vi "Local Test.vi"() -> ()   [LabVIEW 2017]
panel:
  out "String 2":string
  out "Dbl 2":dbl
  out "Boolean 2":bool
  in  "String":string
  in  "Dbl":dbl
  in  "Boolean":bool
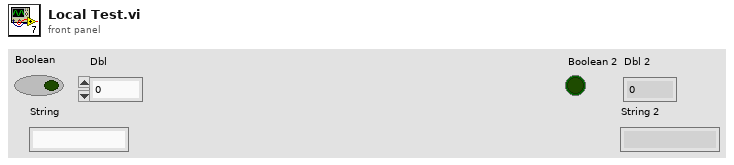
[diagram p1: front panel]
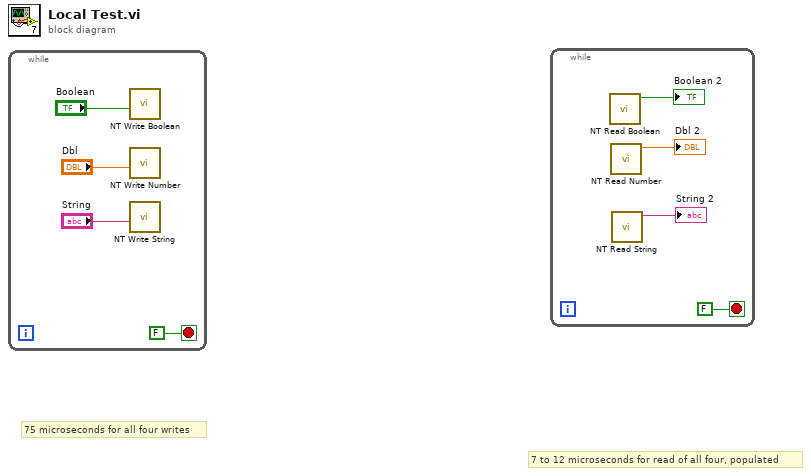
[diagram p0: block diagram]
diagram:
  # "7 to 12 microseconds for read of all four, populated"
  # "75 microseconds for all four writes"
  n1 = while {
    stop <- FALSE stop-if-true
    n2 = call <vilib>:"NT Write Boolean.vi"("Boolean"="Boolean") -> ()  [unwired: 10 in, 1 out]
    n3 = call <vilib>:"NT Write Number.vi"("Numeric"="Dbl") -> ()  [unwired: 10 in, 1 out]
    n4 = call <vilib>:"NT Write String.vi"("String"="String") -> ()  [unwired: 10 in, 1 out]
  }
  n5 = while {
    stop <- FALSE stop-if-true
    n6 = call <vilib>:"NT Read Boolean.vi"() -> ("Boolean"=→"Boolean 2":bool)  [unwired: 10 in, 1 out]
    n7 = call <vilib>:"NT Read Number.vi"() -> ("Numeric"=→"Dbl 2":dbl)  [unwired: 10 in, 1 out]
    n8 = call <vilib>:"NT Read String.vi"() -> ("String"=→"String 2":string)  [unwired: 10 in, 1 out]
  }
